vi "Construct_Bad_Track_For_(101-111)_Point-1.vi"(6 "[IN] Indexes for Jumps":i32[](array[numeric]), 7 "[IN] Number of Co\nnnected Points":i32, 8 "error IN":errorcluster, 9 "[IN] Index of recon\nstructed tracks":i32, 10 "[IN] Clusters for Re\nconstructed Tracks":T1, 11 "[IN] Still connected\ntracks in group":T2) -> (0 "error OUT":errorcluster, 2 "[OUT] Clusters for Re\nconstructed Tracks":T1)   [LabVIEW 2013]
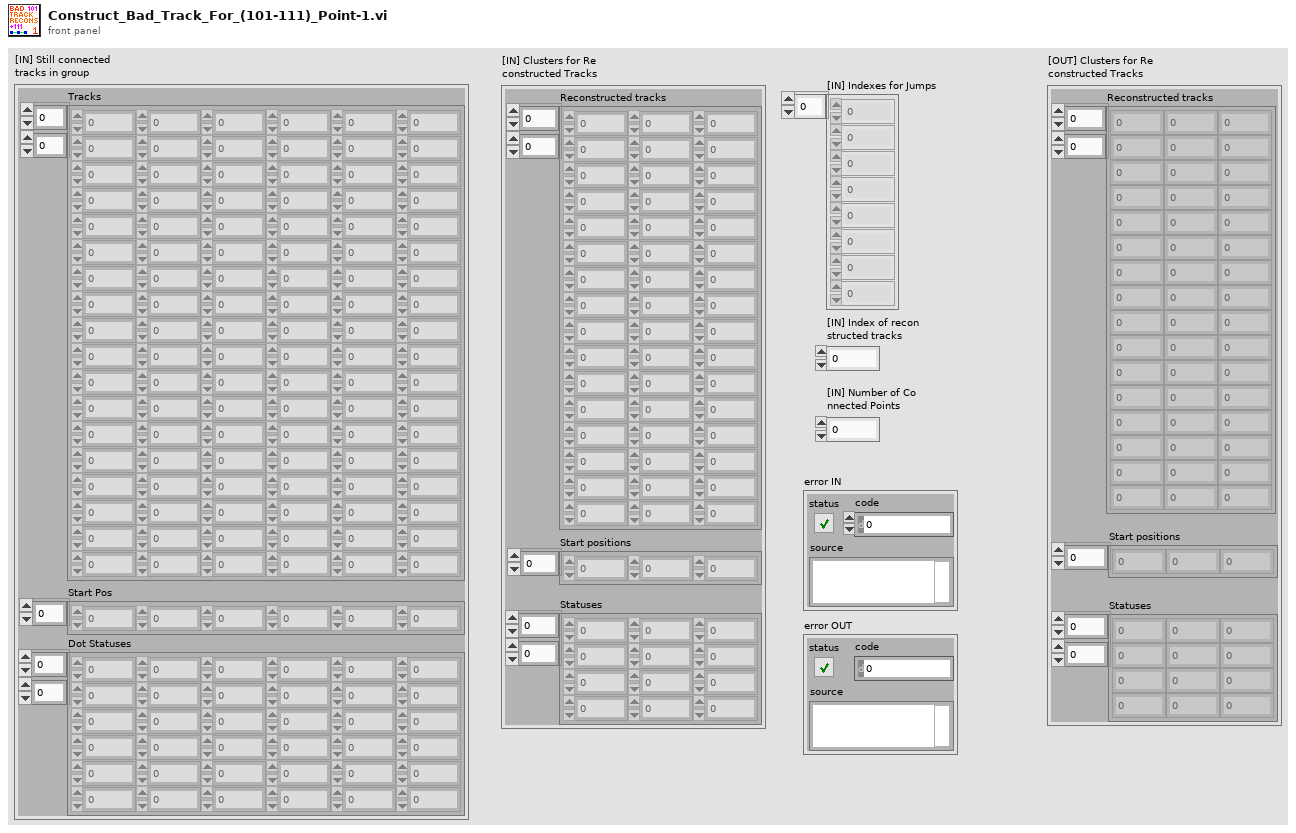
[diagram p1: front panel]
types:
  T1 = cluster{"Reconstructed tracks":dbl[][], "Start positions":i32[], "Statuses":i16[][]}
  T2 = cluster{"Tracks":dbl[][], "Start Pos":i32[], "Dot Statuses":i16[][]}
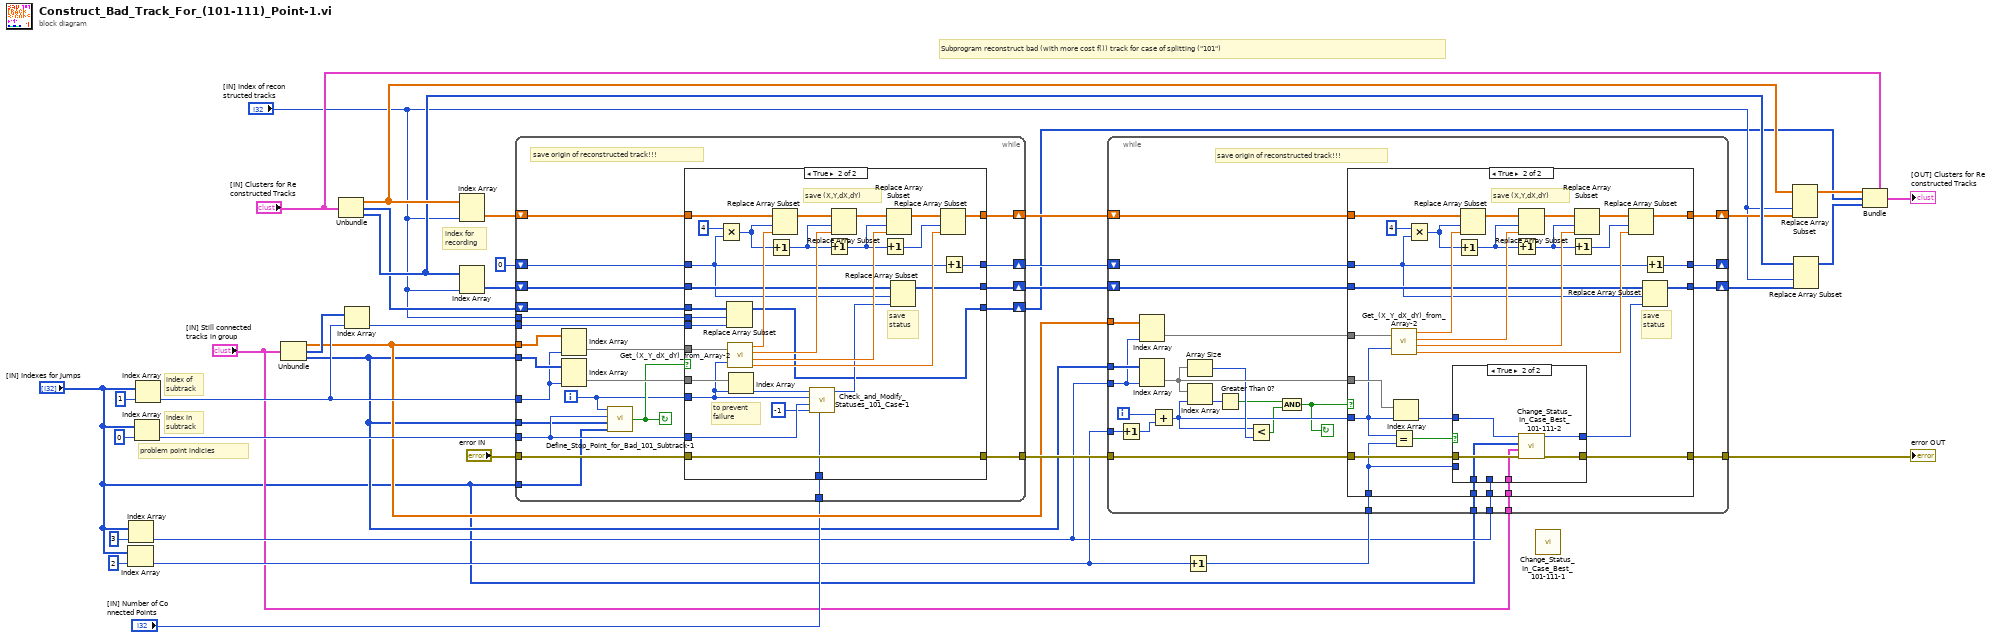
[diagram p0: block diagram]
diagram:
  # "index for\nrecording"
  # "index of\nsubtrack"
  # "index in\nsubtrack"
  # "problem point indicies"
  # "Subprogram reconstruct bad (with more cost f()) track for case of splitting (\"101\")"
  n1 = Index Array(array="[IN] Indexes for Jumps", index=2) -> (element=w9:i32)
  n2 = Index Array(array="[IN] Indexes for Jumps", index=3) -> (element=w3:i32)
  n3 = Index Array(array="[IN] Indexes for Jumps", index=0) -> (element=w27:i32)
  n4 = Index Array(array="[IN] Indexes for Jumps", index=1) -> (element=w30:i32)
  n5 = Unbundle("[IN] Still connected\ntracks in group") -> ("Tracks"=w15:dbl[][], "Start Pos"=w28:i32[], "Dot Statuses"=w10:i16[][])
  n6 = Unbundle("[IN] Clusters for Re\nconstructed Tracks") -> ("Reconstructed tracks"=w34:dbl[][], "Start positions"=w7:i32[], "Statuses"=w33:i16[][])
  n7 = Index Array(array=w28, index=w30) -> (element=w5:i32)
  n8 = Index Array(array=w34, index (col)="[IN] Index of recon\nstructed tracks") -> (element=w26:dbl[])  [unwired: 1 in]
  n9 = Index Array(array=w33, index (col)="[IN] Index of recon\nstructed tracks") -> (element=w25:i16[])  [unwired: 1 in]
  n10 = while {
    tunnel: w27 -> [w43]
    tunnel: w15 -> [w59]
    tunnel: w10 -> [w58]
    tunnel: w30 -> [w57]
    shift-right: [w52] -> w17
    shift-left: w26 -> [w56]
    shift-right: [w50] -> w19
    shift-left: w25 -> [w54]
    shift-right: [w51] -> w18
    shift-left: 0 -> [w53]
    tunnel: "error IN" -> [w49]
    tunnel: [w48] -> w16
    tunnel: "[IN] Number of Co\nnnected Points" -> [w46]
    tunnel: w10 -> [w42]
    tunnel: "[IN] Indexes for Jumps" -> [w41]
    shift-right: [w37] -> w4
    shift-left: w7 -> [w40]
    tunnel: "[IN] Index of recon\nstructed tracks" -> [w39]
    tunnel: w5 -> [w38]
    i -> [w44]
    stop <- w45 continue-if-true
    # "save origin of reconstructed track!!!"
    n11 = Index Array(array=w59, index (col)=w57) -> (element=w55:dbl[])  [unwired: 1 in]
    n12 = Index Array(array=w58, index (col)=w57) -> (element=w47:i16[])  [unwired: 1 in]
    n13 = call "Define_Stop_Point_for_Bad_101_Subtrack-1.vi"("[IN] Indexes for Jumps"=w41, "[IN] Dot Statuses"=w42, "[IN] Index of Mer\nging (\"101\") Point"=w43, "[IN] Current index"=w44) -> ("[OUT] Continue saving points"=w45:bool)
    n14 = case shown="True" w45 {
      tunnel: w56 -> [w64 w93]
      tunnel: w55 -> [_ w95]
      tunnel: w47 -> [_ w94]
      tunnel: w44 -> [_ w73]
      tunnel: w54 -> [w62 w80]
      tunnel: [w62 w79] -> w50
      tunnel: [w64 w78] -> w52
      tunnel: w53 -> [w63 w77]
      tunnel: [w63 w76] -> w51
      tunnel: w49 -> [w61 w75]
      tunnel: [w61 w75] -> w48
      tunnel: w43 -> [_ w72]
      tunnel: w46 -> [_ w71]
      tunnel: w40 -> [w60 w68]
      tunnel: w39 -> [_ w67]
      tunnel: w38 -> [_ w66]
      tunnel: [w60 w65] -> w37
      frame False {
      }
      frame True {
        # "to prevent \nfailure"
        # "save (X,Y,dX,dY)"
        # "save\nstatus"
        n15 = Multiply(x=4, y=w77) -> (x*y=w89:i32)
        n16 = Replace Array Subset(array=w68, new element=w66, index=w67) -> (w65:i32[])
        n17 = call "Get_(X_Y_dX_dY)_from_Array-2.vi"("(X,Y,dX,dY)"=w95, "Index of Displacement"=w73) -> ("X"=w91:dbl, "Y"=w88:dbl, "dX"=w85:dbl, "dY"=w81:dbl)
        n18 = Index Array(array=w94, index=w73) -> (element=w74:i16)
        n19 = Increment(x=w89) -> (x+1=w86:i32)
        n20 = Replace Array Subset(array=w93, new element=w91, index=w89) -> (w90:dbl[])
        n21 = call "Check_and_Modify_Statuses_101_Case-1.vi"("[IN] Number of Co\nnnected Points"=w71, "[IN] Index of Po\nint After \"101\""=-1 ("[IN] Index of Po\nint After \"101\""), "[IN] Index of Pro\nblem \"101\" Point"=w72, "[IN] Current Index"=w73, "[IN] Current Status"=w74) -> ("[OUT] Status"=w70:i16)  [unwired: 4 in]
        n22 = Increment(x=w86) -> (x+1=w84:i32)
        n23 = Replace Array Subset(array=w90, new element=w88, index=w86) -> (w87:dbl[])
        n24 = Increment(x=w84) -> (x+1=w83:i32)
        n25 = Replace Array Subset(array=w87, new element=w85, index=w84) -> (w82:dbl[])
        n26 = Replace Array Subset(array=w80, new element=w70, index=w77) -> (w79:i16[])
        n27 = Replace Array Subset(array=w82, new element=w81, index=w83) -> (w78:dbl[])
        n28 = Increment(x=w77) -> (x+1=w76:i32)
      }
    }
  }
  n29 = Increment(x=w9) -> (x+1=w8:i32)
  n30 = while {
    tunnel: w15 -> [w121]
    tunnel: w10 -> [w120]
    tunnel: w3 -> [w119]
    shift-right: [w114] -> w13
    shift-left: w17 -> [w118]
    shift-right: [w112] -> w12
    shift-left: w19 -> [w116]
    shift-right: [w113] -> _
    shift-left: w18 -> [w115]
    tunnel: w9 -> [w101]
    tunnel: w16 -> [w103]
    tunnel: [w102] -> w11
    tunnel: w8 -> [w99]
    tunnel: w3 -> [w98]
    tunnel: "[IN] Still connected\ntracks in group" -> [w97]
    tunnel: "[IN] Indexes for Jumps" -> [w96]
    i -> [w111]
    stop <- w104 continue-if-true
    # "save origin of reconstructed track!!!"
    n31 = Increment(x=w101) -> (x+1=w100:i32)
    n32 = Index Array(array=w121, index (col)=w119) -> (element=w117:dbl[])  [unwired: 1 in]
    n33 = Index Array(array=w120, index (col)=w119) -> (element=w110:i16[])  [unwired: 1 in]
    n34 = Add(x=w111, y=w100) -> (x+y=w107:i32)
    n35 = Array Size(array=w110) -> (size(s)=w108:i32)
    n36 = Index Array(array=w110, index=w107) -> (element=w109:i16)
    n37 = Greater Than 0?(x=w109) -> (x > 0?=w106:bool)
    n38 = Less?(x=w107, y=w108) -> (x < y?=w105:bool)
    n39 = And(x=w106, y=w105) -> (x .and. y?=w104:bool)
    n40 = case shown="True" w104 {
      tunnel: w118 -> [w125 w154]
      tunnel: w117 -> [_ w155]
      tunnel: w110 -> [_ w136]
      tunnel: w107 -> [_ w134]
      tunnel: w116 -> [w123 w141]
      tunnel: [w123 w140] -> w112
      tunnel: [w125 w139] -> w114
      tunnel: w115 -> [w124 w138]
      tunnel: [w124 w137] -> w113
      tunnel: w103 -> [w122 w135]
      tunnel: [w122 w131] -> w102
      tunnel: w99 -> [_ w128]
      tunnel: w98 -> [_ w129]
      tunnel: w97 -> [_ w127]
      tunnel: w96 -> [_ w126]
      frame False {
      }
      frame True {
        # "save (X,Y,dX,dY)"
        # "save\nstatus"
        n41 = call "Get_(X_Y_dX_dY)_from_Array-2.vi"("(X,Y,dX,dY)"=w155, "Index of Displacement"=w134) -> ("X"=w152:dbl, "Y"=w149:dbl, "dX"=w146:dbl, "dY"=w142:dbl)
        n42 = Equal?(x=w134, y=w128) -> (x = y?=w133:bool)
        n43 = Index Array(array=w136, index=w134) -> (element=w132:i16)
        n44 = Multiply(x=4, y=w138) -> (x*y=w150:i32)
        n45 = case shown="True" w133 {
          tunnel: w135 -> [w156 w163]
          tunnel: w132 -> [w157 w160]
          tunnel: [w156 w162] -> w131
          tunnel: [w157 w161] -> w130
          tunnel: w129 -> [_ _]
          tunnel: w128 -> [_ _]
          tunnel: w127 -> [_ w159]
          tunnel: w126 -> [_ w158]
          frame False {
          }
          frame True {
            n46 = call "Change_Status_In_Case_Best_101-111-2.vi"("error IN"=w163, "[IN] Track group"=w159, "[IN] Indexes for Jumps"=w158, "[IN] Current Status"=w160) -> ("error OUT"=w162:errorcluster, "[OUT] Status of point after 101"=w161:i16)  [unwired: 3 in]
          }
        }
        n47 = Increment(x=w150) -> (x+1=w147:i32)
        n48 = Replace Array Subset(array=w154, new element=w152, index=w150) -> (w151:dbl[])
        n49 = Increment(x=w147) -> (x+1=w145:i32)
        n50 = Replace Array Subset(array=w151, new element=w149, index=w147) -> (w148:dbl[])
        n51 = Increment(x=w145) -> (x+1=w144:i32)
        n52 = Replace Array Subset(array=w148, new element=w146, index=w145) -> (w143:dbl[])
        n53 = Replace Array Subset(array=w143, new element=w142, index=w144) -> (w139:dbl[])
        n54 = Increment(x=w138) -> (x+1=w137:i32)
        n55 = Replace Array Subset(array=w141, new element=w130, index=w138) -> (w140:i16[])
      }
    }
  }
  "error OUT" <- w11
  n56 = call "Change_Status_In_Case_Best_101-111-1.vi"() -> ()  [unwired: 7 in, 2 out]
  n57 = Replace Array Subset(array=w34, new element=w13, index (col)="[IN] Index of recon\nstructed tracks") -> (w22:dbl[][])  [unwired: 1 in]
  n58 = Replace Array Subset(array=w33, new element=w12, index (col)="[IN] Index of recon\nstructed tracks") -> (w23:i16[][])  [unwired: 1 in]
  n59 = Bundle(cluster="[IN] Clusters for Re\nconstructed Tracks", "Reconstructed tracks"=w22, "Start positions"=w4, "Statuses"=w23) -> (→"[OUT] Clusters for Re\nconstructed Tracks":T1)
